vi "SPI_Transaction Example.vi"(5 "Device":i32, 6 "Values to write":u8[](array[numeric])=[1, 0, 0] format="%.0x", 7 "Bus":i32, 8 "error in":errorcluster) -> (0 "error out":errorcluster, 4 "Values read":u8[](array[numeric]) format="%.0x")   [LabVIEW 2014]
doc: "This example demonstrates a simple SPI transaction, simply connect an SPI slave device to the MISO, MOSI, SCK and CE0/CE1 pins. The default bus is 0 and the device is 0 or 1 depending on which CE pin is used."
uses:
  GPIO.lvlib
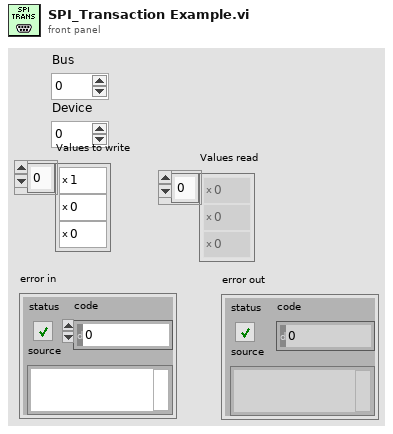
[diagram p1: front panel]
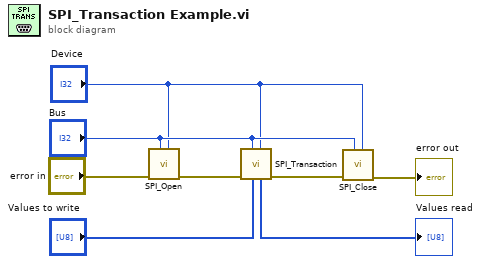
[diagram p0: block diagram]
diagram:
  n1 = call "SPI_Open.vi"("Device"="Device", "Bus"="Bus", "error in"="error in") -> ("error out"=w8:errorcluster)  [unwired: 8 in]
  n2 = call "SPI_Transaction.vi"("Device"="Device", "Values to write"="Values to write", "Bus"="Bus", "error in"=w8) -> ("error out"=w7:errorcluster, "Values read"=→"Values read":u8[])  [unwired: 6 in]
  n3 = call "SPI_Close.vi"("Device"="Device", "Bus"="Bus", "error in"=w7) -> ("error out"=→"error out":errorcluster)  [unwired: 8 in]
